vi "Filter Class Owned Items.vi"(8 "Error In":errorcluster, 10 "Children[]":refnum<vi>[](array[refnum]), 11 "LVClassLibrary In":refnum<vi>) -> (0 "Error Out":errorcluster, 1 "Private Items":refnum<vi>[](array[refnum]), 2 "Non-Private Items":refnum<vi>[](array[refnum]), 3 "LVClassLibrary Out":refnum<vi>)   [LabVIEW 2018, in "Scripts.lvlib"]
uses:
  Scripts.lvlib
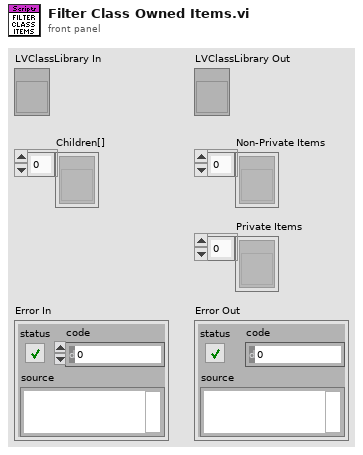
[diagram p1: front panel]
types:
  T1 = enum32{"invalid scope", "public", "private", "protected", "community"}
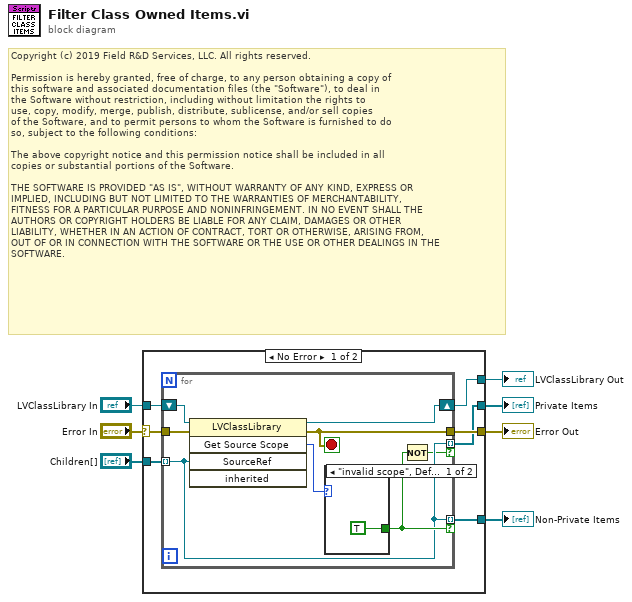
[diagram p0: block diagram]
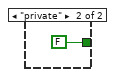
[diagram p2: hidden frame]
diagram:
  # "Copyright (c) 2019 Field R&D Services, LLC. All rights reserved.\n\nPermission is hereby granted, free of charge, to any person obtaining a copy of\nthis software and associated documentation files (the \"Software\"), to deal in\nthe Software without restriction, including without limitation the rights to\nuse, copy, modify, merge, publish, distribute, sublicense, and/or sell copies\nof the Software, and to permit persons to whom the Software is furnished to do\nso, subject to the following conditions:\n\nThe above copyright notice and this permission notice shall be included in all\ncopies or substantial portions of the Software.\n\nTHE SOFTWARE IS PROVIDED \"AS IS\", WITHOUT WARRANTY OF ANY KIND, EXPRESS OR\nIMPLIED, INCLUDING BUT NOT LIMITED TO THE WARRANTIES OF MERCHANTABILITY,\nFITNESS FOR A PARTICULAR PURPOSE AND NONINFRINGEMENT. IN NO EVENT SHALL THE\nAUTHORS OR COPYRIGHT HOLDERS BE LIABLE FOR ANY CLAIM, DAMAGES OR OTHER\nLIABILITY, WHETHER IN AN ACTION OF CONTRACT, TORT OR OTHERWISE, ARISING FROM,\nOUT OF OR IN CONNECTION WITH THE SOFTWARE OR THE USE OR OTHER DEALINGS IN THE\nSOFTWARE."
  n1 = case shown="No Error" "Error In" {
    selector: "Error In" -> [w8 w25]
    tunnel: [w14 _] -> w7
    tunnel: [w13 w26] -> w6
    tunnel: [w12 w25] -> w5
    tunnel: [w11 _] -> w4
    tunnel: "Children[]" -> [w10 _]
    tunnel: "LVClassLibrary In" -> [w9 w26]
    frame No Error {
      n2 = for {
        shift-right: [w21] -> w13
        shift-left: w9 -> [w22]
        tunnel: w10 -> [w16] mode=indexing
        tunnel: w8 -> [w20]
        tunnel: [w19] -> w12
        tunnel: [w16] -> w14 mode=indexing if=w17
        tunnel: [w16] -> w11 mode=indexing if=w15
        stop <- w19 stop-if-true
        n3 = invoke class="LVClassLibrary" method="Get Source Scope"(reference=w22, error in=w20, "SourceRef"=w16) -> (reference out=w21:refnum<vi>, error out=w19:errorcluster, "GetSourceScope"=w18:T1)  [unwired: 2 in, 2 out]
        n4 = case shown="\"invalid scope\", Default" w18 {
          tunnel: [TRUE FALSE] -> w17
          frame "invalid scope", Default {
          }
          frame "private" {
          }
        }
        n5 = Not(x=w17) -> (.not. x?=w15:bool)
      }
    }
    frame Error {
    }
  }
  "Non-Private Items" <- w7
  "LVClassLibrary Out" <- w6
  "Error Out" <- w5
  "Private Items" <- w4
